vi "Pre-Install Custom Action.vi"(10 "Variant":variant) -> (0 "error out":errorcluster)   [LabVIEW 2021]
uses:
  <vilib>/Utility/sysdir.llb/System Directory Type.ctl
  <userlib>/_OpenG.lib/file/file.llb/openg_file.lvlib
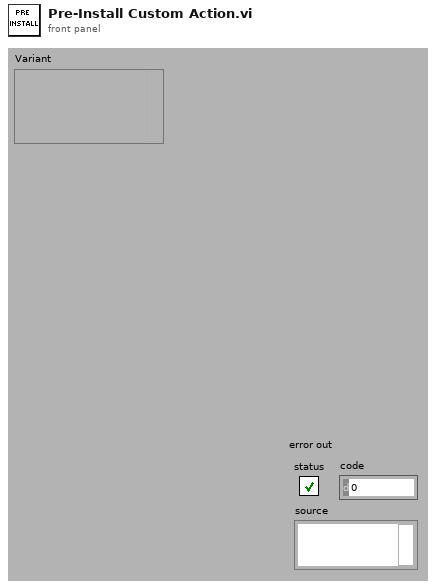
[diagram p1: front panel]
types:
  T1 = enum16{"open", "replace", "create", "open or create", "replace or create", "replace or create with confirmation"}
  T2 = typedef "System Directory Type.ctl" = i32
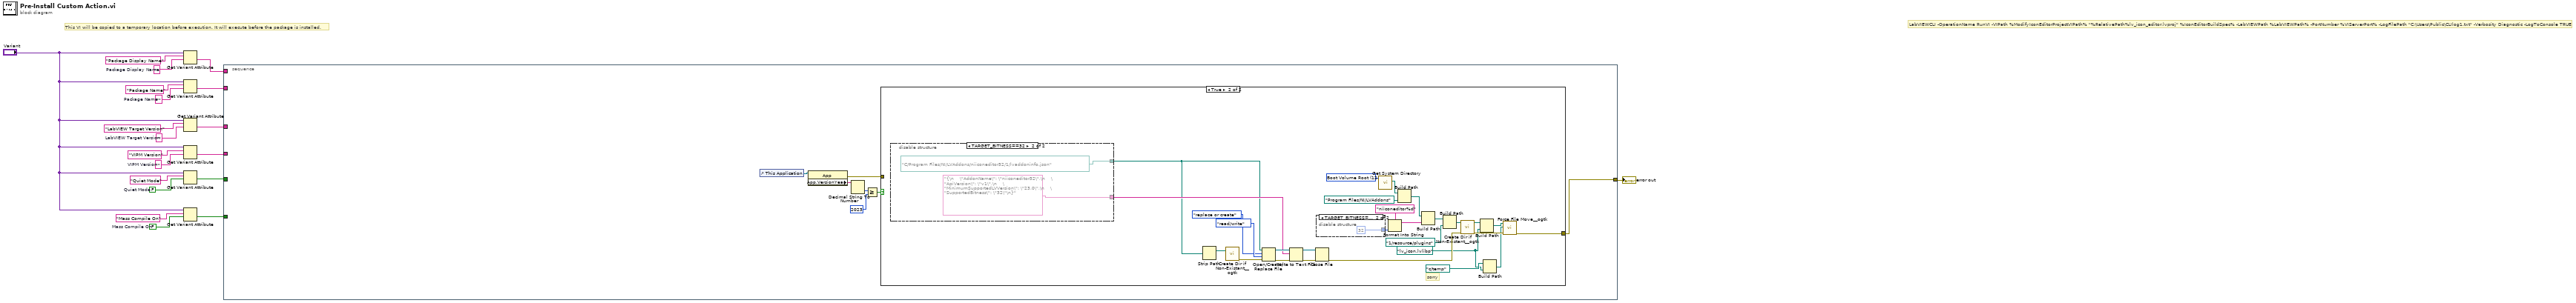
[diagram p0: block diagram]
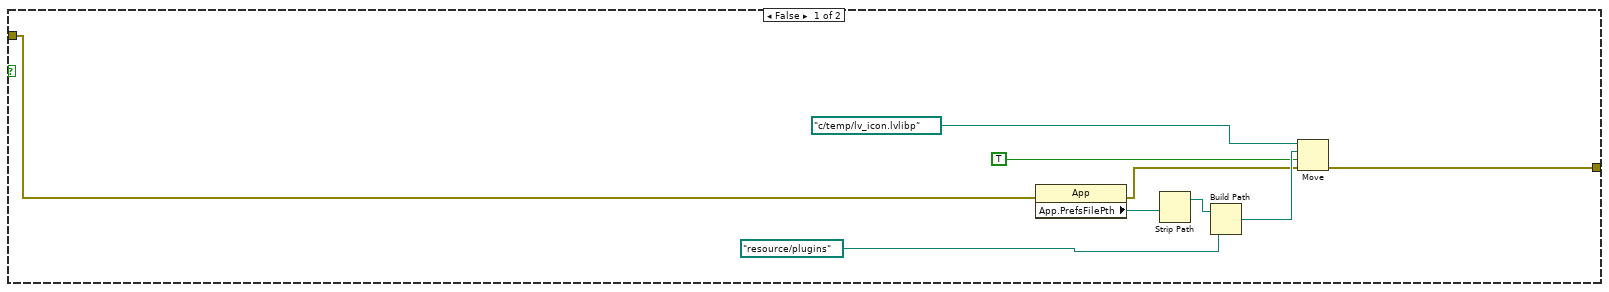
[diagram p2: hidden frame]
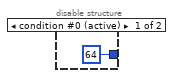
[diagram p3: hidden frame]
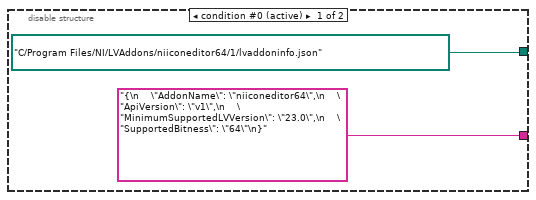
[diagram p4: hidden frame]
diagram:
  w2 = FALSE  # Mass Compile On
  w4 = ""  # Package Display Name
  w11 = FALSE  # Quiet Mode
  w14 = ""  # VIPM Version
  w16 = ""  # LabVIEW Target Version
  w18 = ""  # Package Name
  # "LabVIEWCLI -OperationName RunVI -VIPath %ModifyIconEditorProjectVIPath% \"%RelativePath%lv_icon_editor.lvproj\" %IconEditorBuildSpec% -LabVIEWPath %LabVIEWPath% -PortNumber %VIServerPort% -LogFilePath \"C:\\Users\\Public\\CLIlog1.txt\" -Verbosity Diagnostic -LogToConsole TRUE"
  # "This VI will be copied to a temporary location before execution. It will execute before the package is installed."
  n1 = Get Variant Attribute(Variant="Variant", name="Package Display Name", default value (empty Variant)=w4) -> (value=w10:string)  [unwired: 1 in, 3 out]
  n2 = Get Variant Attribute(Variant="Variant", name="Package Name", default value (empty Variant)=w18) -> (value=w9:string)  [unwired: 1 in, 3 out]
  n3 = Get Variant Attribute(Variant="Variant", name="LabVIEW Target Version", default value (empty Variant)=w16) -> (value=w8:string)  [unwired: 1 in, 3 out]
  n4 = Get Variant Attribute(Variant="Variant", name="VIPM Version", default value (empty Variant)=w14) -> (value=w7:string)  [unwired: 1 in, 3 out]
  n5 = Get Variant Attribute(Variant="Variant", name="Quiet Mode", default value (empty Variant)=w11) -> (value=w6:bool)  [unwired: 1 in, 3 out]
  n6 = Get Variant Attribute(Variant="Variant", name="Mass Compile On", default value (empty Variant)=w2) -> (value=w5:bool)  [unwired: 1 in, 3 out]
  n7 = stacked-sequence {
    tunnel: w10 -> [_]
    tunnel: w9 -> [_]
    tunnel: w8 -> [_]
    tunnel: w7 -> [_]
    tunnel: w6 -> [_]
    tunnel: w5 -> [_]
    tunnel: [w21] -> w1
    frame #0 {
      n8 = control-ref of="This Application"() -> (w27:refnum<vi>)
      n9 = property class="App"(reference=w27) -> (error out=w22:errorcluster, "App.VersionYear"=w26:string)  [unwired: 1 in, 1 out]
      n10 = Decimal String To Number(string=w26) -> (number=w25:i32)  [unwired: 2 in, 1 out]
      n11 = Greater Or Equal?(x=w25, y=2023) -> (x >= y?=w23:bool)
      n12 = case shown="True" w23 {
        tunnel: [w32 w64] -> w21
        tunnel: w22 -> [w29 _]
        frame False {
          n13 = property class="App"(error in=w29) -> (error out=w28:errorcluster, "App.PrefsFilePth"=w36:path)  [unwired: 1 in, 1 out]
          n14 = Strip Path(path=w36) -> (stripped path=w35:path)  [unwired: 1 out]
          n15 = Build Path(base path=w35, name or relative path=path "resource/plugins") -> (appended path=w33:path)
          n16 = Move(source path=path "c:/temp/lv_icon.lvlibp", error in=w28, 9:TRUE ("overwrite (F)"), 10:w33) -> (error out=w32:errorcluster)  [unwired: 1 in, 2 out]
        }
        frame True {
          w40 = path "lv_icon.lvlibp" ("source path")
          w49 = T2 12 items=["User Home"=0, "User Desktop"=1, "User Documents"=2, "User Application Data"=3, "User Preferences"=4, "User Temporary"=5, "Public Documents"=6, "Public Application Data"=7, "Public Preferences"=8, "Public Cache"=13, "System Core Libraries"=9, "System Installed Libraries"=10, "Application Files"=11, "Boot Volume Root"=12] ("system directory type")
          # "sorry"
          n17 = disable-structure shown="TARGET_BITNESS==32" {
            disable-tunnel: [path "C:/Program Files/NI/LVAddons/niiconeditor64/1/lvaddoninfo.json" ("Destination[i] Paths (Absolute)") path "C:/Program Files/NI/LVAddons/niiconeditor32/1/lvaddoninfo.json" ("Destination[i] Paths (Absolute)")] -> w37
            disable-tunnel: ["{\n    \"AddonName\": \"niiconeditor64\",\n    \"ApiVersion\": \"v1\",\n    \"MinimumSupportedLVVersion\": \"23.0\",\n    \"SupportedBitness\": \"64\"\n}" ("Tag Name") "{\n    \"AddonName\": \"niiconeditor32\",\n    \"ApiVersion\": \"v1\",\n    \"MinimumSupportedLVVersion\": \"23.0\",\n    \"SupportedBitness\": \"32\"\n}" ("Tag Name")] -> w57
            frame condition #0 (active) {
            }
            frame condition #1 {
            }
          }
          n18 = Strip Path(path=w37) -> (stripped path=w38:path)  [unwired: 1 out]
          n19 = call <userlib>:"Create Dir if Non-Existant__ogtk.vi"("Directory Path"=w38) -> ("error out"=w44:errorcluster)  [unwired: 8 in, 2 out]
          n20 = Open/Create/Replace File(file path (use dialog)=w37, error in=w44, operation (0:open)=T1."replace or create", access (0:read/write)=enum16{"read/write", "read-only", "write-only"}."read/write") -> (refnum out=w61:refnum<file>, error out=w62:errorcluster)  [unwired: 2 in, 1 out]
          n21 = Write to Text File(file (use dialog)=w61, text=w57, error in=w62) -> (refnum out=w60:refnum<file>, error out=w63:errorcluster)  [unwired: 1 in, 1 out]
          n22 = Close File(refnum=w60, error in=w63) -> (error out=w43:errorcluster)  [unwired: 1 out]
          n23 = disable-structure shown="TARGET_BITNESS==32" {
            disable-tunnel: [64 ("code") 32 ("code")] -> w52
            frame condition #0 (active) {
            }
            frame condition #1 {
            }
          }
          n24 = call <vilib>:"Get System Directory.vi"("system directory type"=w49) -> ("system directory"=w53:path)  [unwired: 10 in]
          n25 = Format Into String(format string="niiconeditor%d", w52) -> (resulting string=w55:string)  [unwired: 2 in, 1 out]
          n26 = Build Path(base path=w53, name or relative path=path "Program Files/NI/LVAddons") -> (appended path=w54:path)
          n27 = Build Path(base path=w54, name or relative path=w55) -> (appended path=w56:path)
          n28 = Build Path(base path=w56, name or relative path=path "1/resource/plugins") -> (appended path=w47:path)
          n29 = call <userlib>:"Create Dir if Non-Existant__ogtk.vi"("error in (no error)"=w43, "Directory Path"=w47) -> ("error out"=w45:errorcluster, "dup Directory Path"=w46:path)  [unwired: 7 in, 1 out]
          n30 = Build Path(base path=w46, name or relative path=w40) -> (appended path=w42:path)
          n31 = Build Path(base path=path "c:/temp" ("source path"), name or relative path=w40) -> (appended path=w39:path)
          n32 = call <userlib>:"Force File Move__ogtk.vi"("error in (no error)"=w45, "source"=w39, "target"=w42) -> ("error out"=w64:errorcluster)  [unwired: 3 in, 1 out]
        }
      }
    }
  }
  "error out" <- w1
